vi "Get Events.vi"(11 "Analyzing Dialog View in":refnum<class "Analyzing Dialog View.lvclass">) -> (2 "Events":T1, 3 "Analyzing Dialog View out":refnum<class "Analyzing Dialog View.lvclass">)   [LabVIEW 2013, in "Analyzing Dialog View.lvlib" / "Analyzing Dialog View.lvclass"]
uses:
  Analyzing Dialog View.lvclass
  Typedef/Events.ctl
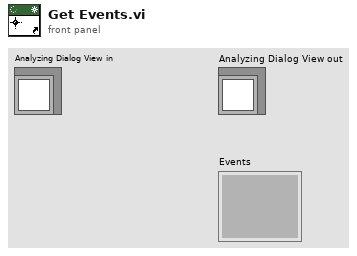
[diagram p1: front panel]
types:
  T1 = typedef "Analyzing Dialog View.lvlib/Analyzing Dialog View.lvclass/Events.ctl" = cluster{}
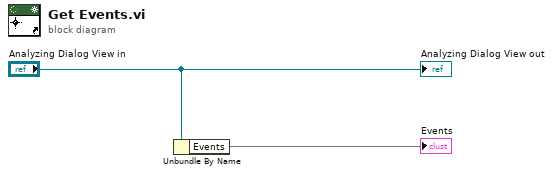
[diagram p0: block diagram]
diagram:
  n1 = Unbundle By Name("Analyzing Dialog View in") -> ("Events"=→"Events")
  "Analyzing Dialog View out" <- "Analyzing Dialog View in"
